vi "Calculate defocus.vi"(8 "error in (no error)":errorcluster, 11 "Cascade in":refnum<class "Cascade.lvclass">) -> (0 "error out":errorcluster, 1 "fine?":bool, 2 "translation out":dbl[unit], 3 "Cascade out":refnum<class "Cascade.lvclass">)   [LabVIEW 2012, in "Cascade.lvclass"]
uses:
  Cascade.lvclass
  Cascade.lvclass/Cascade.ctl
  <vilib>/vision/NI_Vision_Development_Module.lvlib
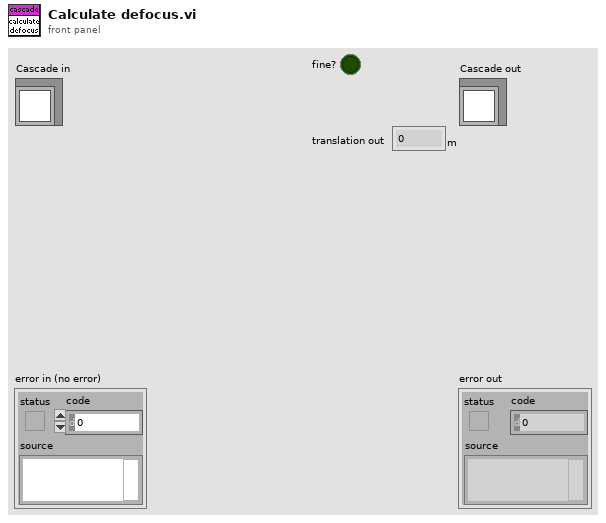
[diagram p1: front panel]
types:
  T1 = typedef "IMAQ Image.ctl" = refnum<image>
  T2 = cluster{"histogram":u32[], "Minimal Value":sgl, "Maximal Value":sgl, "Starting Value":sgl, "Interval Width":sgl, "Mean Value":sgl, "Standard  Variation":sgl, "Area (pixels)":i32}
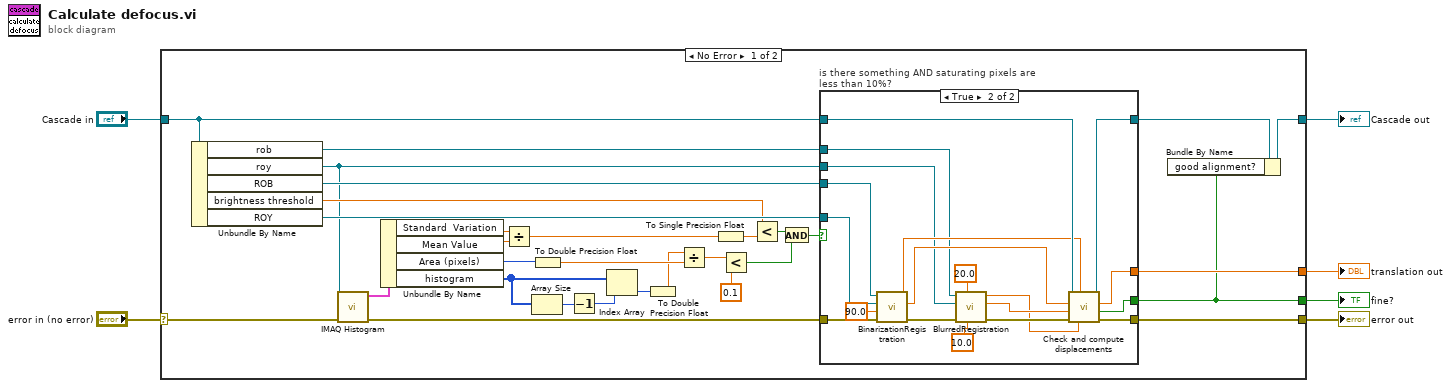
[diagram p0: block diagram]
diagram:
  n1 = case shown="No Error" "error in (no error)" {
    selector: "error in (no error)" -> [w28 w59]
    tunnel: [w34 w59] -> w5
    tunnel: [w8 w58] -> w3
    tunnel: "Cascade in" -> [w32 w58]
    tunnel: [w33 _] -> w1
    tunnel: [w7 _] -> w2
    frame No Error {
      n2 = Unbundle By Name(w32) -> ("rob"=w35:T1, "roy"=w26:T1, "ROB"=w36:T1, "brightness threshold"=w30:sgl, "ROY"=w31:T1)
      n3 = call "IMAQ Histogram"("error in (no error)"=w28, "Image"=w26) -> ("error out"=w27:errorcluster, "Histogram Report"=w25:T2)  [unwired: 8 in]
      n4 = Unbundle By Name(w25) -> ("Standard  Variation"=w24:sgl, "Mean Value"=w23:sgl, "Area (pixels)"=w18:i32, "histogram"=w21:u32[])
      n5 = Divide(x=w24, y=w23) -> (x/y=w22:sgl)
      n6 = Array Size(array=w21) -> (size(s)=w20:i32)
      n7 = To Double Precision Float(number=w18) -> (double precision float=w16:dbl)
      n8 = Decrement(x=w20) -> (x-1=w19:i32)
      n9 = Index Array(array=w21, index=w19) -> (element=w17:u32)
      n10 = To Double Precision Float(number=w17) -> (double precision float=w14:dbl)
      n11 = Divide(x=w14, y=w16) -> (x/y=w15:dbl)
      n12 = To Single Precision Float(number=w22) -> (single precision float=w29:sgl)
      n13 = Less?(x=w15, y=0.1) -> (x < y?=w12:bool)
      n14 = Less?(x=w30, y=w29) -> (x < y?=w11:bool)
      n15 = And(x=w11, y=w12) -> (x .and. y?=w10:bool)
      n16 = case "is there something AND saturating pixels are less than 10%?" shown="True" w10 {
        tunnel: w36 -> [_ w43]
        tunnel: w26 -> [_ w41]
        tunnel: w35 -> [_ w42]
        tunnel: [w38 w56] -> w9
        tunnel: [w37 w54] -> w34
        tunnel: [_ w53] -> w33
        tunnel: [_ w52] -> w7
        tunnel: w32 -> [w38 w49]
        tunnel: w31 -> [_ w40]
        tunnel: w27 -> [w37 w44]
        frame False {
        }
        frame True {
          n17 = call "BinarizationRegistration.vi"("error in"=w44, "threshold percentage"=90.0, "Roy"=w40, "Rob"=w43) -> ("error out"=w57:errorcluster, "y translation"=w46:dbl, "x translation"=w45:dbl)  [unwired: 4 in, 1 out]
          n18 = call "BlurredRegistration.vi"("small sigma"=sgl 10.0, "large sigma"=sgl 20.0, "error in"=w57, "roy"=w41, "rob"=w42) -> ("error out"=w55:errorcluster, "y displacement"=w48:dbl, "x displacement"=w47:dbl)  [unwired: 3 in, 1 out]
          n19 = call-dynamic "Check and compute displacements.vi"("x pixel displacement 2"=w47, "x pixel displacement 1"=w45, "error in (no error)"=w55, "y pixel displacement 2"=w48, "y pixel displacement 1"=w46, "Cascade in"=w49) -> ("error out"=w54:errorcluster, "fine?"=w52:bool, "translation out"=w53:dbl[unit], "Cascade out"=w56:refnum<class "Cascade.lvclass">)  [unwired: 2 in]
        }
      }
      n20 = Bundle By Name(cluster=w9, "good alignment?"=w7) -> (w8:refnum<class "Cascade.lvclass">)
    }
    frame Error {
    }
  }
  "error out" <- w5
  "Cascade out" <- w3
  "fine?" <- w2
  "translation out" <- w1
